vi "RD Analog IO Channel Node Set.vi"(7 "CalArray":u8[](array[numeric]), 8 "error in (no error)":errorcluster caption="错误输入（无错误）", 9 "value":dbl, 10 "ch":i32, 11 "handle":u64) -> (0 "error out":errorcluster caption="错误输出", 2 "function return":i32, 3 "handle out":u64, 5 "CalArray out":u8[](array[numeric]))   [LabVIEW 2018, in "InstrumentsPlayground.lvlib"]
doc: "CLIFFAPI int CliffAnalogIOChannelNodeSet(FT_HANDLE handle,int ch,double value) ;\nCLIFFAPI int CliffAnalogIOChannelNodeSet(FT_HANDLE handle,int ch,double value,int* CalArray) ;"
uses:
  InstrumentsPlayground.lvlib
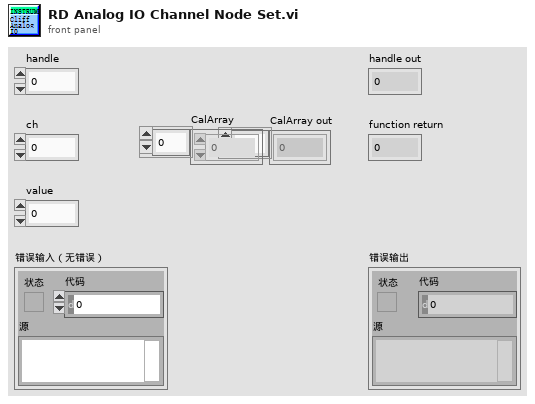
[diagram p1: front panel]
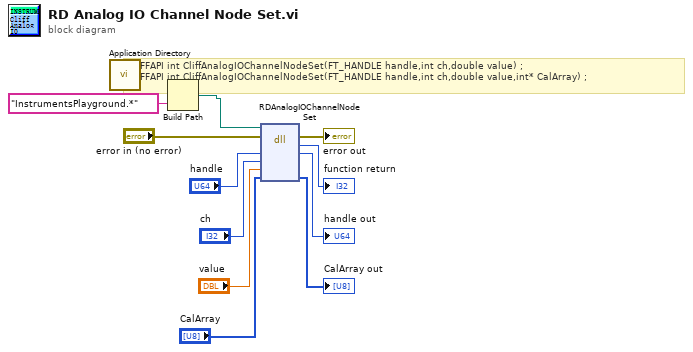
[diagram p0: block diagram]
diagram:
  # "CLIFFAPI int CliffAnalogIOChannelNodeSet(FT_HANDLE handle,int ch,double value) ;\nCLIFFAPI int CliffAnalogIOChannelNodeSet(FT_HANDLE handle,int ch,double value,int* CalArray) ;"
  n1 = call <vilib>:"Application Directory.vi"() -> ("Application Directory"=w3:path)
  n2 = Build Path(base path=w3, name or relative path="InstrumentsPlayground.*" ("名称或相对路径")) -> (appended path=w2:path)
  n3 = dll-call lib="E:/Work/YZCourse_Xtext/Cliff/API/IPLabView lib/InstrumentsPlayground.*" fn="RDAnalogIOChannelNodeSet"(path in=w2, error in="error in (no error)", "handle"="handle", "ch"="ch", "value"="value", "CalArray"="CalArray") -> (error out=→"error out":errorcluster, "返回类型"=→"function return":i32, "handle"=→"handle out":u64, "CalArray"=→"CalArray out":u8[])  [unwired: 3 in, 1 out]
